vi "Draw Mouse.vi"(7 "Grid Size (10)":i32=10, 10 "Direction":T1, 11 "Position":T2) -> (3 "Picture":picture)   [LabVIEW 2020, in "App.lvlib" / "MazeUI.lvclass"]
uses:
  MazeUI.lvclass
  Maze/Position.ctl
  Maze/Direction.ctl
  Maze/Maze.lvlib
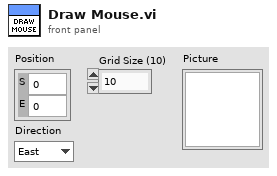
[diagram p1: front panel]
types:
  T1 = typedef "Maze.lvlib/Direction.ctl" = enum8{"East", "North", "West", "South"}
  T2 = typedef "Maze.lvlib/Position.ctl" = cluster{"S":i32, "E":i32}
  T3 = cluster{"Width":u16, "Style":enum32{"Solid", "Dash", "Dot", "DashDot", "DashDotDot"}}
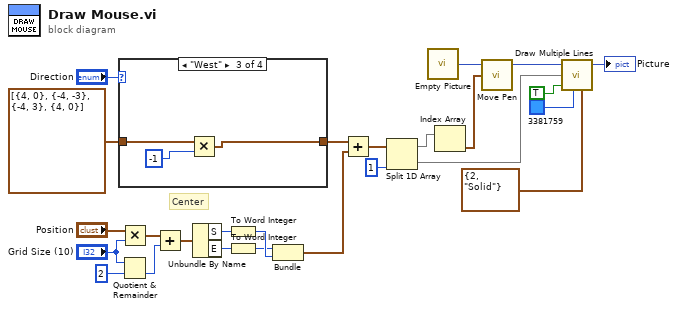
[diagram p0: block diagram]
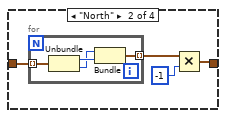
[diagram p3: hidden frame]
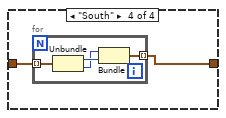
[diagram p4: hidden frame]
diagram:
  # "Center"
  n1 = case shown="\"West\"" "Direction" {
    tunnel: cluster{i16, i16}[] [{4, 0}, {-4, -3}, {-4, 3}, {4, 0}] -> [w26 w30 w37 w39]
    tunnel: [w26 w27 w35 w38] -> w10
    frame "East" {
    }
    frame "North" {
      n2 = for {
        tunnel: w30 -> [w34] mode=indexing
        tunnel: [w31] -> w29 mode=indexing
        n3 = Unbundle(w34) -> (w33:i16, w32:i16)
        n4 = Bundle(w32, w33) -> (w31:cluster{i16, i16})  [unwired: 1 in]
      }
      n5 = Multiply(x=w29, y=i16 -1) -> (x*y=w27:cluster{i16, i16}[])
    }
    frame "West" {
      n6 = Multiply(x=w37, y=i16 -1) -> (x*y=w35:cluster{i16, i16}[])
    }
    frame "South" {
      n7 = for {
        tunnel: w39 -> [w43] mode=indexing
        tunnel: [w40] -> w38 mode=indexing
        n8 = Unbundle(w43) -> (w42:i16, w41:i16)
        n9 = Bundle(w41, w42) -> (w40:cluster{i16, i16})  [unwired: 1 in]
      }
    }
  }
  n10 = Multiply(x="Position", y="Grid Size (10)") -> (x*y=w22:T2)
  n11 = Quotient & Remainder(x="Grid Size (10)", y=2) -> (floor(x/y)=w21:i32)  [unwired: 1 out]
  n12 = Add(x=w22, y=w21) -> (x+y=w20:T2)
  n13 = Unbundle By Name(w20) -> ("S"=w16:i32, "E"=w17:i32)
  n14 = To Word Integer(number=w16) -> (16bit integer=w15:i16)
  n15 = To Word Integer(number=w17) -> (16bit integer=w14:i16)
  n16 = Bundle(w14, w15) -> (w8:cluster{i16, i16})  [unwired: 1 in]
  n17 = Add(x=w10, y=w8) -> (x+y=w7:cluster{i16, i16}[])
  n18 = Split 1D Array(array=w7, index=1) -> (first subarray=w3:cluster{i16, i16}[], second subarray=w1:cluster{i16, i16}[])
  n19 = call "Empty Picture"() -> ("empty picture"=w4:picture)
  n20 = Index Array(array=w3) -> (element=w2:cluster{i16, i16})  [unwired: 1 in]
  n21 = call <vilib>:"Move Pen.vi"("new position"=w2, "picture"=w4) -> ("new picture"=w5:picture)  [unwired: 3 in]
  n22 = call <vilib>:"Draw Multiple Lines.vi"("picture"=w5, "line endpoints"=w1, "fill?(F)"=TRUE, "color(black)"=u32 3381759, "pen"=T3 {"Width"=2, "Style"=enum."Solid"}) -> ("new picture"=→"Picture":picture)  [unwired: 4 in]
